vi "Get All Instrument Value(SubVI).vi"(11 "输出簇 2":T1={"initialize"=enum."SR830", "6221"={"6221 Resource"="GPIB0::24::INSTR", "Delta status"=FALSE, "电流"=0.0}, "SR830+6221"={"source"=0, "阻抗"=0.0, "量程入 4"=0, "量程入 3"=0, "量程入 2"=0, "量程入 1"=0, "SR830 2"=FALSE, "SR830 3"=FALSE, "SR830 4"=FALSE, "SR830 1"=FALSE, "VISA 1"="", "VISA 2"="", "VISA 3"="", "VISA 4"="", "Reserve 1"=0, "Reserve 2"=-1, "Reserve 3"=-1, "Reserve 4"=-1, "量程"=enum."量程每次测量会判定"}, "2400"={"2400"=FALSE, "VISA"=""}, "ch"={"ch"=[], "current"=[], "change?"=[], "holding current\nwhen change ch?"=FALSE}, "Instrument"={"335 Resource"="GPIB0::24::INSTR", "Input (0:A)"=0, "Instrument Type"=enum."SVSM", "quantum design"=refnum, "Heater Output (1:1)"=1, "semaphore"=refnum, "TCP master instance"=refnum, "335 Status"=refnum, "M24C Resource"="GPIB0::24::INSTR", "4G supply"="GPIB0::24::INSTR", "Temp Status 24C"=refnum, "4g supply status"=refnum, "Temp"=refnum, "9T信号"=refnum}, "Aborting"=refnum, "数据文件"=refnum} {"Instrument"."Input (0:A)" items=["A", "B"]; "Instrument"."Heater Output (1:1)" items=["1"=1, "2"=2]; "SR830+6221"."Reserve 4" items=["Auto Reserve"=-1, "High Reserve"=0, "Normal"=1, "Low Noise"=2]; "SR830+6221"."Reserve 3" items=["Auto Reserve"=-1, "High Reserve"=0, "Normal"=1, "Low Noise"=2]; "SR830+6221"."Reserve 2" items=["Auto Reserve"=-1, "High Reserve"=0, "Normal"=1, "Low Noise"=2]; "SR830+6221"."Reserve 1" items=["量程每次测量会判定", "量程不变为设定值"]; "SR830+6221"."source" items=["SR830 1", "SR830 2", "SR830 3", "SR830 4"]}) -> (2 "数组":dbl[](array[numeric]))   [LabVIEW 2019, in "Get value.lvlib"]
uses:
  Get value.lvlib
  config.ctl
  <vilib>/NI/Modbus Library/API/Master/Modbus Master.lvclass
  initialize.ctl
  Instrument.ctl
  Instrument Type.ctl
  lib/QDInstrument.dll
  335 state.ctl
  lib/Lake Shore 335/Lake Shore 335.lvlib
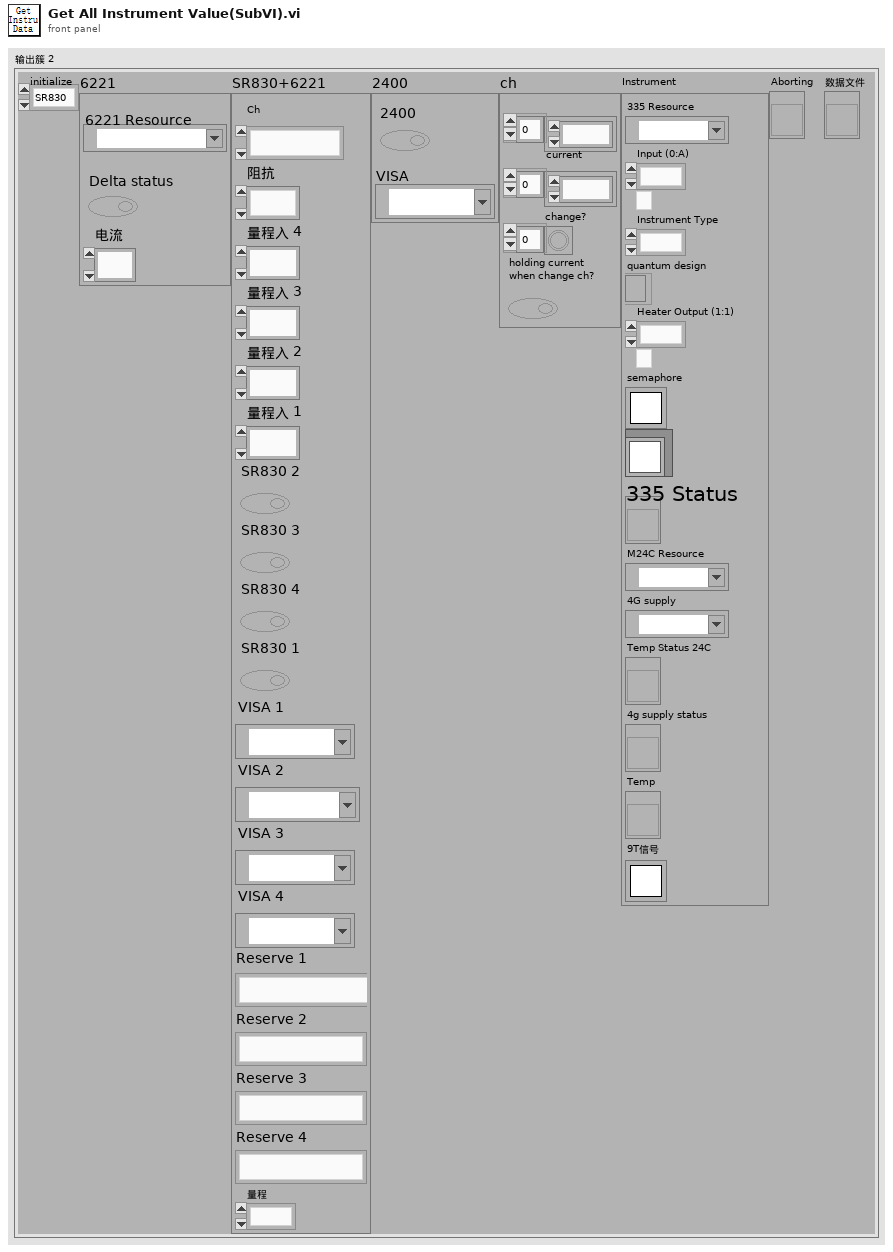
[diagram p1: front panel]
types:
  T1 = typedef "config.ctl" = cluster{"initialize":T2, "6221":cluster{"6221 Resource":refnum<visa-resource-name>, "Delta status":bool, "电流":dbl}, "SR830+6221":cluster{"source":u16, "阻抗":dbl, "量程入 4":i32, "量程入 3":i32, "量程入 2":i32, "量程入 1":i32, "SR830 2":bool, "SR830 3":bool, "SR830 4":bool, "SR830 1":bool, "VISA 1":refnum<visa-resource-name>, "VISA 2":refnum<visa-resource-name>, "VISA 3":refnum<visa-resource-name>, "VISA 4":refnum<visa-resource-name>, "Reserve 1":i16, "Reserve 2":i16, "Reserve 3":i16, "Reserve 4":i16, "量程":enum16{"量程每次测量会判定", "量程不变为设定值"}}, "2400":cluster{"2400":bool, "VISA":refnum<visa-resource-name>}, "ch":cluster{"ch":i32[], "current":dbl[], "change?":bool[], "holding current\nwhen change ch?":bool}, "Instrument":T3, "Aborting":refnum<vi>, "数据文件":refnum<vi>}
  T2 = typedef "initialize.ctl" = enum16{"SR830", "keithley6221-SR830", "Delta", "Delta-tunnelling", "keithley6221-2182-DC"}
  T3 = typedef "Instrument.ctl" = cluster{"335 Resource":refnum<visa-resource-name>, "Input (0:A)":u16, "Instrument Type":T4, "quantum design":refnum<k24>, "Heater Output (1:1)":u16, "semaphore":T5, "TCP master instance":refnum<class "Modbus Master.lvclass">, "335 Status":refnum<vi>, "M24C Resource":refnum<visa-resource-name>, "4G supply":refnum<visa-resource-name>, "Temp Status 24C":refnum<vi>, "4g supply status":refnum<vi>, "Temp":refnum<vi>, "9T信号":T5}
  T4 = typedef "Instrument Type.ctl" = enum16{"PPMS", "VersaLab", "DynaCool", "SVSM", "PPMS-Rotate", "Lakeshore335", "9T mag"}
  T5 = typedef "Semaphore RefNum" = refnum<k1>
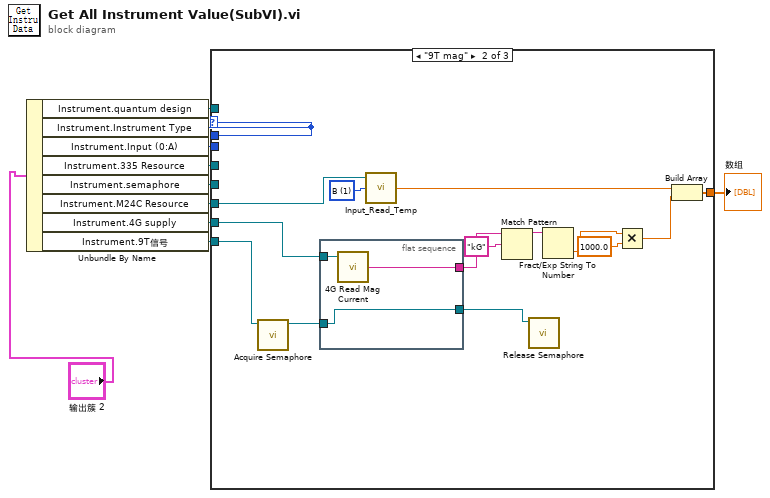
[diagram p0: block diagram]
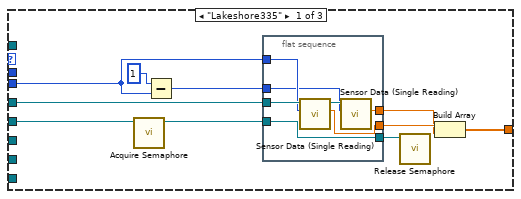
[diagram p2: hidden frame]
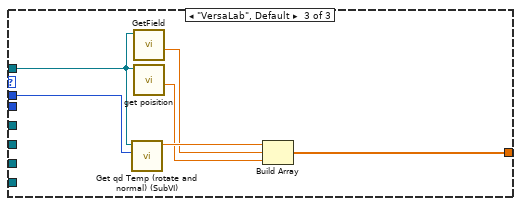
[diagram p3: hidden frame]
diagram:
  n1 = Unbundle By Name("输出簇 2") -> ("Instrument.quantum design"=w9:refnum<k24>, "Instrument.Instrument Type"=w8:T4, "Instrument.Input (0:A)"=w6:u16, "Instrument.335 Resource"=w7:refnum<visa-resource-name>, "Instrument.semaphore"=w5:T5, "Instrument.M24C Resource"=w3:refnum<visa-resource-name>, "Instrument.4G supply"=w4:refnum<visa-resource-name>, "Instrument.9T信号"=w1:T5)
  n2 = case shown="\"9T mag\"" w8 {
    tunnel: w8 -> [_ _ w50]
    tunnel: [w14 w31 w46] -> w10
    tunnel: w9 -> [_ _ w45]
    tunnel: w7 -> [w20 _ _]
    tunnel: w6 -> [w19 _ _]
    tunnel: w5 -> [w11 _ _]
    tunnel: w4 -> [_ w41 _]
    tunnel: w3 -> [_ w40 _]
    tunnel: w1 -> [_ w30 _]
    frame "Lakeshore335" {
      n3 = call <vilib>:"Acquire Semaphore.vi"("semaphore"=w11) -> ("semaphore out"=w13:T5)  [unwired: 4 in, 2 out]
      n4 = Subtract(x=u16 1, y=w19) -> (x-y=w17:u16)
      n5 = flat-sequence {
        tunnel: w20 -> [w27]
        tunnel: w19 -> [w25]
        tunnel: w17 -> [w24]
        tunnel: [w23] -> w16
        tunnel: [w22] -> w15
        tunnel: w13 -> [w21]
        tunnel: [w21] -> w12
        frame #0 {
          n6 = call "Sensor Data (Single Reading).vi"("Input (0:A)"=w25, "VISA resource name"=w27) -> ("Sensor Data"=w23:dbl, "VISA resource name out"=w26:refnum<visa-resource-name>)  [unwired: 7 in, 1 out]
          n7 = call "Sensor Data (Single Reading).vi"("Input (0:A)"=w24, "VISA resource name"=w26) -> ("Sensor Data"=w22:dbl)  [unwired: 7 in, 2 out]
        }
      }
      n8 = call <vilib>:"Release Semaphore.vi"("semaphore"=w12) -> ()  [unwired: 5 in, 2 out]
      n9 = Build Array(w16, w15) -> (w14:dbl[])
    }
    frame "9T mag" {
      w39 = u8 1 items=["A", "B", "C", "D"] ("Input")
      n10 = call <vilib>:"Acquire Semaphore.vi"("semaphore"=w30) -> ("semaphore out"=w29:T5)  [unwired: 4 in, 2 out]
      n11 = flat-sequence {
        tunnel: w41 -> [w44]
        tunnel: [w43] -> w37
        tunnel: w29 -> [w42]
        tunnel: [w42] -> w28
        frame #0 {
          n12 = call "4G Read Mag Current.vi"("VISA session"=w44) -> ("response out"=w43:string)  [unwired: 2 in, 2 out]
        }
      }
      n13 = call "Input_Read_Temp.vi"("Input"=w39, "VISA In"=w40) -> ("Temperature"=w38:dbl)  [unwired: 1 in, 2 out]
      n14 = Match Pattern(string=w37, regular expression="kG" ("正则表达式")) -> (before substring=w35:string)  [unwired: 1 in, 3 out]
      n15 = call <vilib>:"Release Semaphore.vi"("semaphore"=w28) -> ()  [unwired: 5 in, 2 out]
      n16 = Fract/Exp String To Number(string=w35) -> (number=w34:dbl)  [unwired: 3 in, 1 out]
      n17 = Multiply(x=w34, y=1000.0) -> (x*y=w32:dbl)
      n18 = Build Array(w38, w32) -> (w31:dbl[])
    }
    frame "VersaLab", Default {
      n19 = call "Get qd Temp (rotate and normal) (SubVI).vi"("Instrument Type"=w50, ".NET引用句柄输入"=w45) -> ("Temperature"=w49:dbl)  [unwired: 9 in]
      n20 = call "GetField.vi"("Instrument Ref In"=w45) -> ("Field"=w48:dbl)  [unwired: 4 in, 4 out]
      n21 = call "get poisition.vi"("Instrument Ref In"=w45) -> ("Position"=w47:dbl)  [unwired: 4 in, 2 out]
      n22 = Build Array(w49, w48, w47) -> (w46:dbl[])
    }
  }
  "数组" <- w10
